vi "SQLite insert values.vi"(5 "是否创建唯一键":bool, 6 "columns  INFO":string[](array[string]), 7 "数组":variant[][](array[variant]), 8 "错误输入（无错误）":errorcluster, 9 "columns外部输入":T1, 10 "database":string="database1.db", 11 "Tabe Name":string) -> (0 "错误输出":errorcluster)   [LabVIEW 2016, in "SQLite Lib.lvlib"]
uses:
  SQLite Lib.lvlib
  <userlib>/_LVST/sqlite_api/Core/Utils/SQLite_Pragma Cmd.ctl
  <userlib>/_LVST/sqlite_api/Core/Tables/SQLite_Create Table.vi
  <userlib>/_LVST/sqlite_api/Core/Tables/SQLite_List Columns.vi
  <userlib>/_LVST/sqlite_api/Core/Tables/SQLite_Add Column.vi
  <userlib>/_LVST/sqlite_api/Core/Insert/SQLite_Insert Table.vi
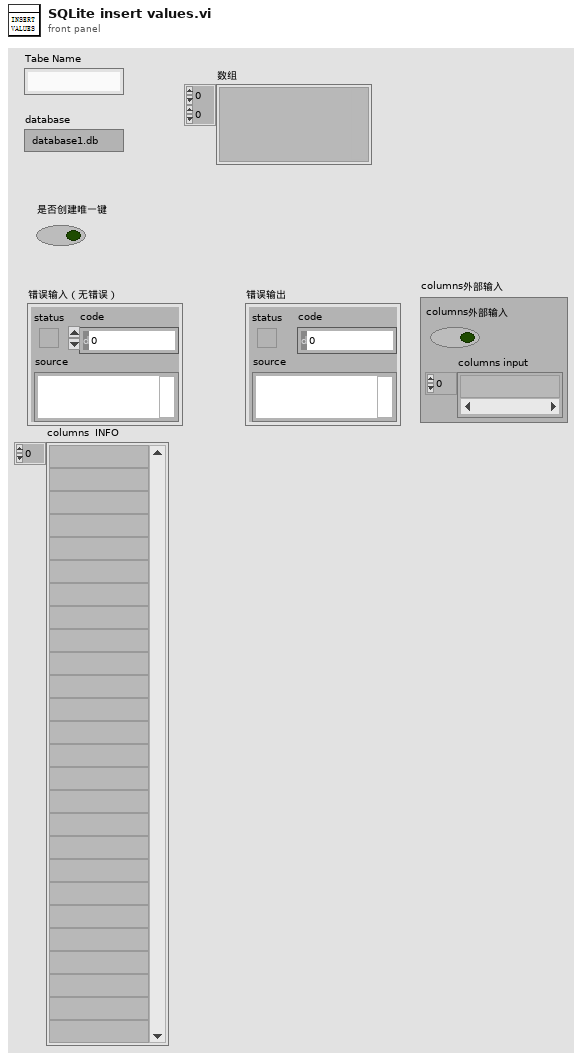
[diagram p1: front panel]
types:
  T1 = cluster{"columns外部输入":bool, "columns input":string[]}
  T2 = typedef "SQLite_Pragma Cmd.ctl" = u16
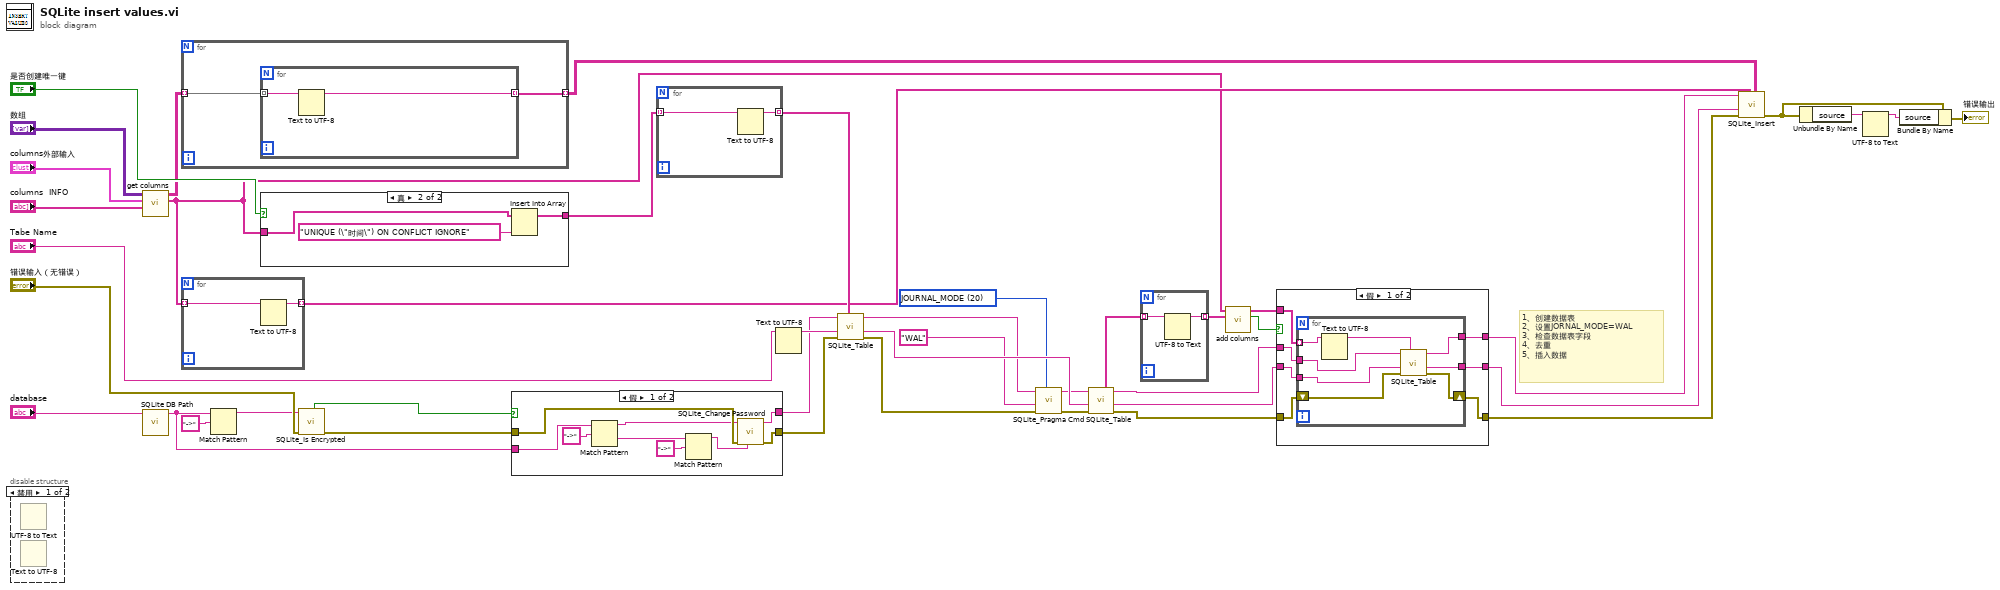
[diagram p0: block diagram]
diagram:
  w31 = T2 20 items=["AUTO_VACUUM", "AUTOMATIC_INDEX", "CACHE_SIZE", "CASE_SENSITIVE_LIKE", "COLLATION_LIST", "COMPILE_OPTIONS", "COUNT_CHANGES", "DATABASE_LIST", "DEFAULT_CACHE_SIZE", "EMPTY_RESULT_CALLBACKS", "ENCODING", "FOREIGN_KEY_LIST", "FOREIGN_KEYS", "FREELIST_COUNT", "FULL_COLUMN_NAMES", "FULLFSYNC", "INCREMENTAL_VACUUM", "INDEX_INFO", "INDEX_LIST", "INTEGRITY_CHECK", "JOURNAL_MODE", "JOURNAL_SIZE_LIMIT", "KEY", "LEGACY_FILE_FORMAT", "LOCKING_MODE", "MAX_PAGE_COUNT", "PAGE_COUNT", "PAGE_SIZE", "QUICK_CHECK", "READ_UNCOMMITTED", "REKEY", "RECURSIVE_TRIGGERS", "REVERSE_UNORDERED_SELECTS", "SCHEMA_VERSION", "SECURE_DELETE", "SHORT_COLUMN_NAMES", "SYNCHRONOUS", "TABLE_INFO", "TEMP_STORE", "TEMP_STORE_DIRECTORY", "USER_VERSION", "WAL_AUTOCHECKPOINT", "WAL_CHECKPOINT", "BUSY_TIMEOUT"] ("Cmd")
  # "1、创建数据表\n2、设置JORNAL_MODE=WAL\n3、检查数据表字段\n4、去重\n5、插入数据"
  n1 = disable-structure shown="禁用" {
    frame Disabled {
      n2 = UTF-8 to Text() -> ()  [unwired: 3 in, 2 out]
      n3 = Text to UTF-8() -> ()  [unwired: 3 in, 2 out]
    }
    frame Enabled {
    }
  }
  n4 = call "get columns.vi"("columns  INFO"="columns  INFO", "columns外部输入"="columns外部输入", "数组"="数组") -> ("columns output"=w9:string[], "data"=w12:string[][])  [unwired: 7 in]
  n5 = call "SQLite DB Path.vi"("database"="database") -> ("Path out"=w2:string)  [unwired: 10 in]
  n6 = for {
    tunnel: w12 -> [w44] mode=indexing
    tunnel: [w43] -> w11 mode=indexing
    n7 = for {
      tunnel: w44 -> [w46] mode=indexing
      tunnel: [w45] -> w43 mode=indexing
      n8 = Text to UTF-8(11:w46) -> (3:w45:string)  [unwired: 2 in, 1 out]
    }
  }
  n9 = for {
    tunnel: w9 -> [w48] mode=indexing
    tunnel: [w47] -> w13 mode=indexing
    n10 = Text to UTF-8(11:w48) -> (3:w47:string)  [unwired: 2 in, 1 out]
  }
  n11 = Match Pattern(string=w2, regular expression="->" ("正则表达式")) -> (before substring=w3:string)  [unwired: 1 in, 3 out]
  n12 = case shown="真" "是否创建唯一键" {
    tunnel: [w49 w52] -> w17
    tunnel: w9 -> [w49 w51]
    frame False {
    }
    frame True {
      n13 = Insert Into Array(array=w51, new element="UNIQUE (\"时间\") ON CONFLICT IGNORE" ("新元素/子数组")) -> (w52:string[])  [unwired: 1 in]
    }
  }
  n14 = call <userlib>:"SQLite_Is Encrypted.vi"("error in (no error)"="错误输入（无错误）", "Path"=w3) -> ("error out"=w7:errorcluster, "Encrypted?"=w6:bool)  [unwired: 6 in, 1 out]
  n15 = case shown="假" w6 {
    tunnel: w7 -> [w61 w62]
    tunnel: w2 -> [w54 w63]
    tunnel: [w53 w63] -> w5
    tunnel: [w60 w62] -> w4
    frame False {
      n16 = Match Pattern(string=w54, regular expression="->" ("正则表达式")) -> (before substring=w55:string, after substring=w58:string)  [unwired: 1 in, 2 out]
      n17 = Match Pattern(string=w58, regular expression="->" ("正则表达式")) -> (before substring=w56:string)  [unwired: 1 in, 3 out]
      n18 = call <userlib>:"SQLite_Change Password.vi"("New Password (Empty to remove)"=w56, "error in (no error)"=w61, "DB Path"=w55) -> ("error out"=w60:errorcluster, "Modified DB Path Out"=w53:string)  [unwired: 7 in]
    }
    frame True {
    }
  }
  n19 = for {
    tunnel: w17 -> [w65] mode=indexing
    tunnel: [w64] -> w16 mode=indexing
    n20 = Text to UTF-8(11:w65) -> (3:w64:string)  [unwired: 2 in, 1 out]
  }
  n21 = Text to UTF-8(11:"Tabe Name") -> (3:w18:string)  [unwired: 2 in, 1 out]
  n22 = call-poly <userlib>:"SQLite_Table.vi"("DB Path"=w5, "Table Name"=w18, "error in (no error)"=w4, "Columns"=w16) -> ("DB Path Out"=w29:string, "Table Name Out"=w32:string, "error out"=w27:errorcluster)  [unwired: 4 in]
  n23 = call <userlib>:"SQLite_Pragma Cmd.vi"("Cmd"=w31, "error in (no error)"=w27, "Value"="WAL" ("multi-line string"), "DB Path"=w29) -> ("error out"=w26:errorcluster, "DB Path Out"=w28:string)  [unwired: 3 in, 1 out]
  n24 = call-poly <userlib>:"SQLite_Table.vi"("DB Path"=w28, "Table Name"=w32, "error in (no error)"=w26) -> ("Columns"=w15:string[], "DB Path Out"=w39:string, "Table Name Out"=w38:string, "error out"=w37:errorcluster)  [unwired: 4 in]
  n25 = for {
    tunnel: w15 -> [w67] mode=indexing
    tunnel: [w66] -> w14 mode=indexing
    n26 = UTF-8 to Text(11:w67) -> (3:w66:string)  [unwired: 2 in, 1 out]
  }
  n27 = call "add columns.vi"("Old Col"=w14, "New Col"=w9) -> ("为空？"=w33:bool, "add col"=w40:string[])  [unwired: 8 in]
  n28 = case shown="假" w33 {
    tunnel: w40 -> [w74 _]
    tunnel: w39 -> [w73 w83]
    tunnel: w38 -> [w72 w84]
    tunnel: w37 -> [w68 w85]
    tunnel: [w71 w83] -> w36
    tunnel: [w70 w84] -> w35
    tunnel: [w69 w85] -> w34
    frame False {
      n29 = for {
        tunnel: w74 -> [w76] mode=indexing
        tunnel: w73 -> [w82]
        tunnel: w72 -> [w81]
        tunnel: [w80] -> w71
        tunnel: [w79] -> w70
        shift-right: [w78] -> w69
        shift-left: w68 -> [w77]
        n30 = Text to UTF-8(11:w76) -> (3:w75:string)  [unwired: 2 in, 1 out]
        n31 = call-poly <userlib>:"SQLite_Table.vi"("DB Path"=w82, "Table Name"=w81, "error in"=w77, "Field Declaration"=w75) -> ("DB Path Out"=w80:string, "Table Name Out"=w79:string, "error out"=w78:errorcluster)  [unwired: 4 in]
      }
    }
    frame True {
    }
  }
  n32 = call-poly <userlib>:"SQLite_Insert.vi"("Value Table"=w11, "Column"=w13, "error in"=w34, "Tabe Name"=w35, "DB Path"=w36) -> ("error out"=w25:errorcluster)  [unwired: 1 in, 3 out]
  n33 = Unbundle By Name(w25) -> ("source"=w24:string)
  n34 = UTF-8 to Text(11:w24) -> (3:w21:string)  [unwired: 2 in, 1 out]
  n35 = Bundle By Name(cluster=w25, "source"=w21) -> (→"错误输出":errorcluster)
